vi "Programmatically Smite.vi"() -> ()   [LabVIEW 2017]
doc: "A demonstration of programmatically smiting a zombie (enabled legacy code) at a grave (Diagram Disable Structure) using the Eulogy Toolkit API. The zombie is returned to a corpse in the block diagram for the Smite - Simple.vi example."
uses:
  <vilib>/Utility/traverseref.llb/VI Scripting - Traverse.lvlib
  <vilib>/Utility/traverseref.llb/TRef TravTarget.ctl
  Toolkit/Toolkit.lvlib
panel:
  in  "Stop Button":bool
  # "Overview: Demonstrates programmatically smite a zombie using the Smite - Simple.vi as a target\nInstructions:\n1. Run the VI\n2. The Smite - Simple.vi's block diagram will be displayed automatically\n3. The Zombie (enabled legacy) frame of the grave will be smited (disabled) and the Spirit (refactored) frame will be enabled.\n4. Click the Stop button\n5. The programmatic smite will be undone to leave the Smite - Simple.vi example in its original state."
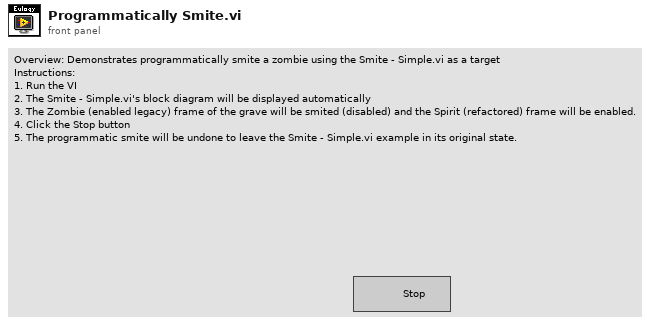
[diagram p1: front panel]
types:
  T1 = typedef "TRef TravTarget.ctl" = enum16{"FP", "BD", "Other"}
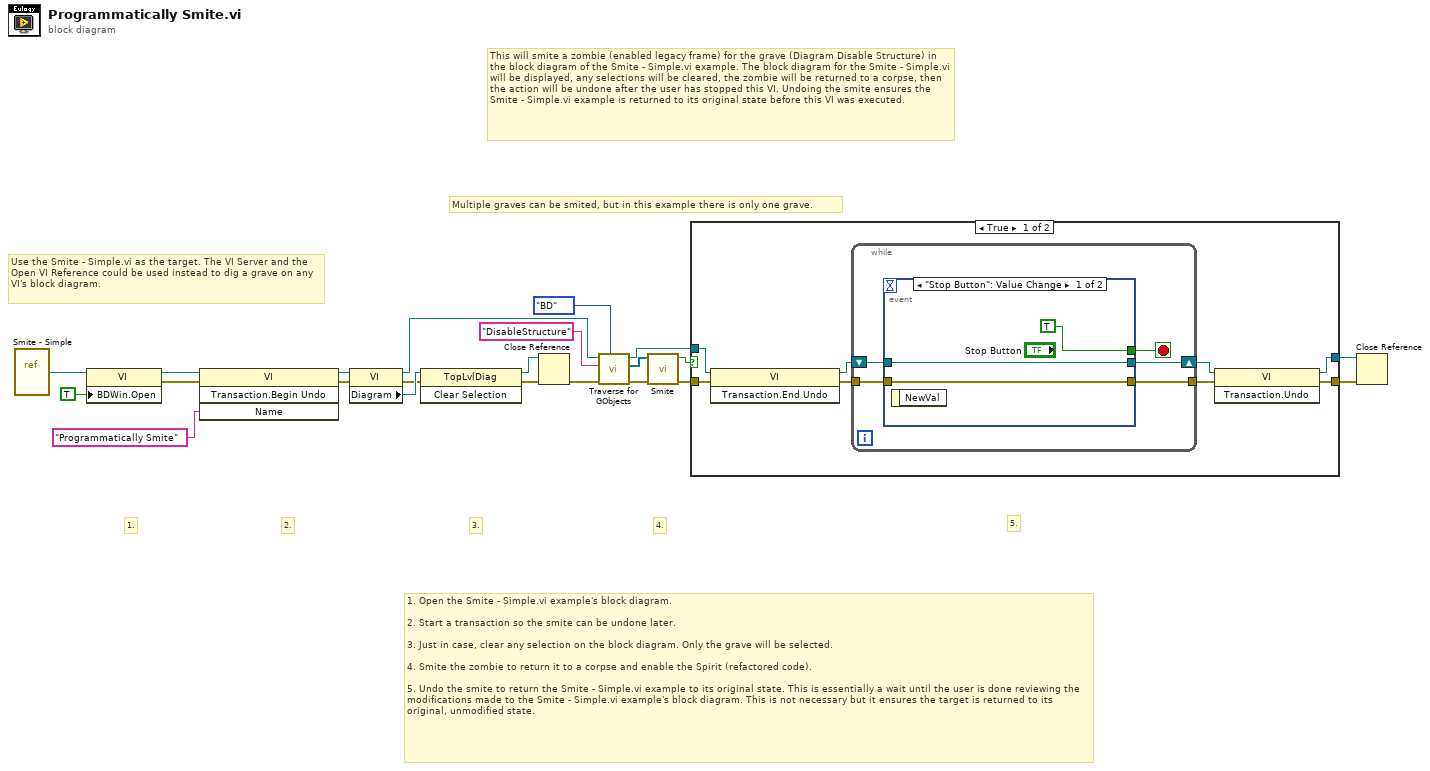
[diagram p0: block diagram]
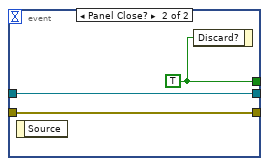
[diagram p2: hidden frame]
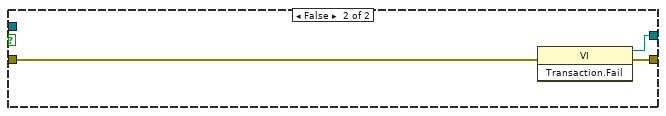
[diagram p3: hidden frame]
diagram:
  # "Multiple graves can be smited, but in this example there is only one grave."
  # "This will smite a zombie (enabled legacy frame) for the grave (Diagram Disable Structure) in the block diagram of the Smite - Simple.vi example. The block diagram for the Smite - Simple.vi will be displayed, any selections will be cleared, the zombie will be returned to a corpse, then the action will be undone after the user has stopped this VI. Undoing the smite ensures the Smite - Simple.vi example is returned to its original state before this VI was executed."
  # "Use the Smite - Simple.vi as the target. The VI Server and the Open VI Reference could be used instead to dig a grave on any VI's block diagram."
  # "1. Open the Smite - Simple.vi example's block diagram.\n\n2. Start a transaction so the smite can be undone later.\n\n3. Just in case, clear any selection on the block diagram. Only the grave will be selected.\n\n4. Smite the zombie to return it to a corpse and enable the Spirit (refactored code).\n\n5. Undo the smite to return the Smite - Simple.vi example to its original state. This is essentially a wait until the user is done reviewing the modifications made to the Smite - Simple.vi example's block diagram. This is not necessary but it ensures the target is returned to its original, unmodified state."
  # "5."
  # "4."
  # "3."
  # "2."
  # "1."
  n1 = vi-ref "Smite - Simple.vi"() -> (w18:refnum<vi>)
  n2 = property class="VI"(reference=w18, "BDWin.Open"=TRUE ("Block Diagram Window:Open")) -> (reference out=w17:refnum<vi>, error out=w15:errorcluster)  [unwired: 1 in]
  n3 = invoke class="VI" method="Transaction.Begin Undo"(reference=w17, error in=w15, "Name"="Programmatically Smite") -> (reference out=w11:refnum<vi>, error out=w10:errorcluster)  [unwired: 1 in, 2 out]
  n4 = property class="VI"(reference=w11, error in=w10) -> (reference out=w5:refnum<vi>, error out=w8:errorcluster, "Diagram"=w9:refnum<vi>)
  n5 = invoke class="TopLvlDiag" method="Clear Selection"(reference=w9, error in=w8) -> (reference out=w6:refnum<vi>, error out=w7:errorcluster)  [unwired: 1 in, 1 out]
  n6 = Close Reference(reference=w6, error in (no error)=w7) -> (error out=w4:errorcluster)
  n7 = call <vilib>:"Traverse for GObjects.vi"("Traverse Target"=TRef_TravTarget."BD", "error in (no error)"=w4, "Class Name"="DisableStructure", "VI Refnum"=w5) -> ("error out"=w12:errorcluster, "References"=w13:refnum<vi>[], "dup VI Refnum"=w3:refnum<vi>)  [unwired: 4 in, 1 out]
  n8 = call "Smite.vi"("Error In"=w12, "Graves"=w13) -> ("Error Out"=w2:errorcluster, "Change Made?"=w1:bool)  [unwired: 8 in]
  n9 = case shown="True" w1 {
    tunnel: [w27 w44] -> w20
    tunnel: [w28 w43] -> w19
    tunnel: w3 -> [w24 _]
    tunnel: w2 -> [w23 w42]
    frame True {
      n10 = invoke class="VI" method="Transaction.End Undo"(reference=w24, error in=w23) -> (reference out=w30:refnum<vi>, error out=w26:errorcluster)  [unwired: 1 in, 1 out]
      n11 = while {
        shift-right: [w34] -> w29
        shift-left: w30 -> [w35]
        tunnel: w26 -> [w33]
        tunnel: [w32] -> w25
        stop <- w31 stop-if-true
        n12 = event shown="[0] \"Stop Button\": Value Change" {
          selector: _ -> [_ _]
          dyn-events: _ -> [_ _]
          timeout: _ -> [_ _]
          tunnel: w35 -> [w38 w41]
          tunnel: [w38 w41] -> w34
          tunnel: w33 -> [w37 w40]
          tunnel: [w37 w40] -> w32
          tunnel: [TRUE w39] -> w31
          event "Stop Button": Value Change {
            n13 = event-data() -> ()  [unwired: 1 in, 1 out]
          }
          event Panel Close? {
            w39 = TRUE
            n14 = event-data() -> ()  [unwired: 1 in, 1 out]
            n15 = event-data("Discard?"=w39) -> ()  [unwired: 1 in, 1 out]
          }
        }
      }
      n16 = invoke class="VI" method="Transaction.Undo"(reference=w29, error in=w25) -> (reference out=w28:refnum<vi>, error out=w27:errorcluster)  [unwired: 1 in, 1 out]
    }
    frame False {
      n17 = invoke class="VI" method="Transaction.Fail"(error in=w42) -> (reference out=w43:refnum<vi>, error out=w44:errorcluster)  [unwired: 2 in, 1 out]
    }
  }
  n18 = Close Reference(reference=w19, error in (no error)=w20) -> ()  [unwired: 1 out]
